vi "getImageArray.vi"(8 "error in (no error)":errorcluster, 11 "CameraAcquisitor.lvclass in":refnum<class "CameraAcquisitor.lvclass">) -> (0 "error out":errorcluster, 2 "Image Array":u32[](array[numeric]), 3 "CameraAcquisitor.lvclass out":refnum<class "CameraAcquisitor.lvclass">)   [LabVIEW 2011, in "Hardware.lvlib" / "Channels.lvlib" / "CameraAcquisitor.lvclass"]
uses:
  CameraAcquisitor.lvclass
  CameraAcquisitor.lvclass/CameraAcquisitor.ctl
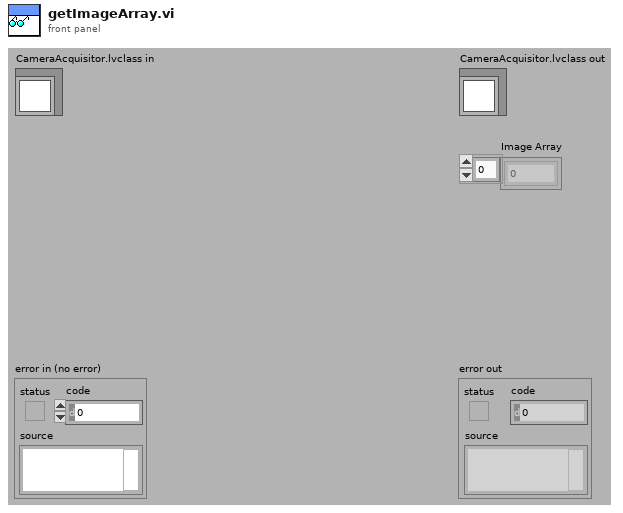
[diagram p1: front panel]
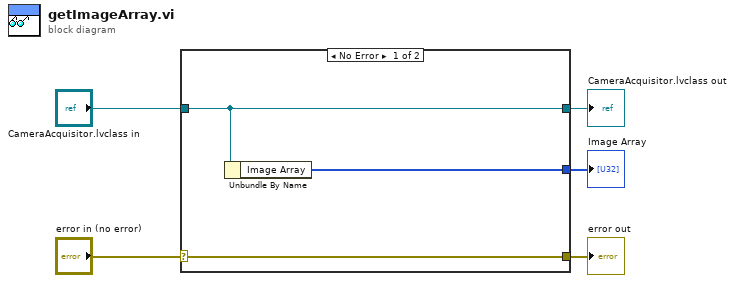
[diagram p0: block diagram]
diagram:
  n1 = case shown="No Error" "error in (no error)" {
    selector: "error in (no error)" -> [w8 w9]
    tunnel: [w8 w9] -> w4
    tunnel: [w7 w10] -> w2
    tunnel: "CameraAcquisitor.lvclass in" -> [w7 w10]
    tunnel: [w6 _] -> w1
    frame No Error {
      n2 = Unbundle By Name(w7) -> ("Image Array"=w6:u32[])
    }
    frame Error {
    }
  }
  "error out" <- w4
  "CameraAcquisitor.lvclass out" <- w2
  "Image Array" <- w1
